vi "getTasksFromList.vi"(8 "error in (no error)":errorcluster, 10 "User Selection":i32[](array[numeric]), 11 "BuildServer in":refnum<class "BuildServer.lvclass">) -> (0 "error out":errorcluster, 2 "Selected Tasks":refnum<class "Task.lvclass">[](array[class]))   [LabVIEW 2017, in "BuildServer.lvlib" / "BuildServer.lvclass"]
uses:
  BuildServer.lvclass
  Classes/Task Interface/Task/Task.lvclass
  BuildServer.lvclass/BuildServer.ctl
  <vilib>/Ekim/LUT/LUT/LUT.lvclass
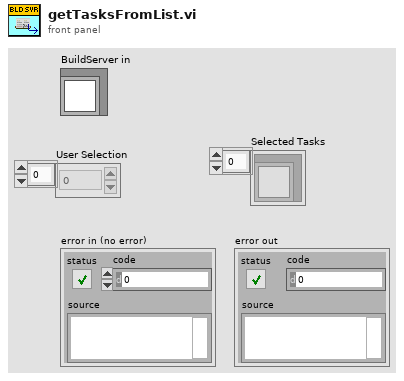
[diagram p1: front panel]
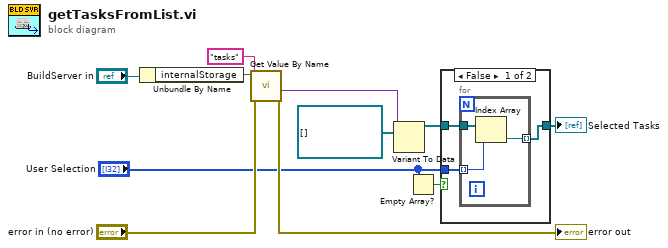
[diagram p0: block diagram]
diagram:
  n1 = Unbundle By Name("BuildServer in") -> ("internalStorage"=w7:refnum<class "LUT.lvclass">)
  n2 = call <vilib>:"Get Value By Name.vi"("error in (no error)"="error in (no error)", "Name"="tasks", "LUT in"=w7) -> ("error out"=→"error out":errorcluster, "Value"=w8:variant)  [unwired: 5 in, 2 out]
  n3 = Variant To Data(type=refnum<class "Task.lvclass">[] [] ("Selected Tasks"), Variant=w8) -> (data=w4:refnum<class "Task.lvclass">[])  [unwired: 1 in, 1 out]
  n4 = Empty Array?(array="User Selection") -> (empty?=w1:bool)
  n5 = case shown="False" w1 {
    tunnel: "User Selection" -> [w14 _]
    tunnel: w4 -> [w13 w18]
    tunnel: [w12 w18] -> w3
    frame False {
      n6 = for {
        tunnel: w14 -> [w16] mode=indexing
        tunnel: w13 -> [w17]
        tunnel: [w15] -> w12 mode=indexing
        n7 = Index Array(array=w17, index=w16) -> (element=w15:refnum<class "Task.lvclass">)
      }
    }
    frame True {
    }
  }
  "Selected Tasks" <- w3
